vi "Name Save File.vi"(11 "Selected File":path) -> (2 "Name":string, 3 "stripped path":path)   [LabVIEW 2021]
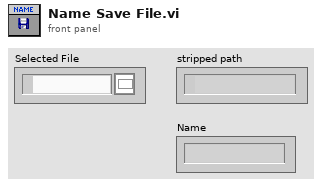
[diagram p1: front panel]
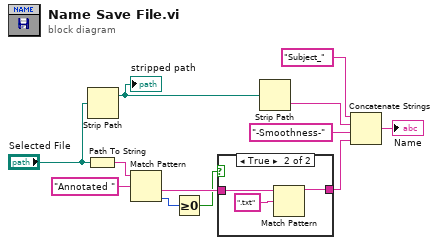
[diagram p0: block diagram]
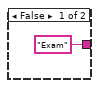
[diagram p2: hidden frame]
diagram:
  n1 = Path To String(path="Selected File") -> (string=w7:string)
  n2 = Strip Path(path="Selected File") -> (stripped path=w11:path)  [unwired: 1 out]
  "stripped path" <- w11
  n3 = Match Pattern(string=w7, regular expression="Annotated ") -> (after substring=w9:string, offset past match=w1:i32)  [unwired: 1 in, 2 out]
  n4 = Greater Or Equal To 0?(x=w1) -> (x >= 0?=w2:bool)
  n5 = case shown="True" w2 {
    tunnel: ["Exam" w16] -> w10
    tunnel: w9 -> [_ w14]
    frame False {
    }
    frame True {
      n6 = Match Pattern(string=w14, regular expression=".txt") -> (before substring=w16:string)  [unwired: 1 in, 3 out]
    }
  }
  n7 = Strip Path(path=w11) -> (name=w12:string)  [unwired: 1 out]
  n8 = Concatenate Strings("Subject_" ("string"), w12, "-Smoothness-" ("string"), w10) -> (→"Name":string)
